vi "decodeStream.vi"(8 "error in (no error)":errorcluster, 9 "beginIndex":i32, 10 "binary stream":u8[](array[numeric]), 11 "tBSONDocumentElement in":refnum<class "tBSONDocumentElement.lvclass">) -> (0 "error out":errorcluster, 1 "endIndex":i32, 2 "binary stream out":u8[](array[numeric]), 3 "tBSONDocumentElement out":refnum<class "tBSONDocumentElement.lvclass">)   [LabVIEW 2013, in "BSON.lvlib" / "tBSONDocumentElement.lvclass"]
uses:
  tBSONDocumentElement.lvclass
  tBSONElement/tBSONElement.lvclass
  setValue.vi
  tBSONDocument/tBSONDocument.lvclass
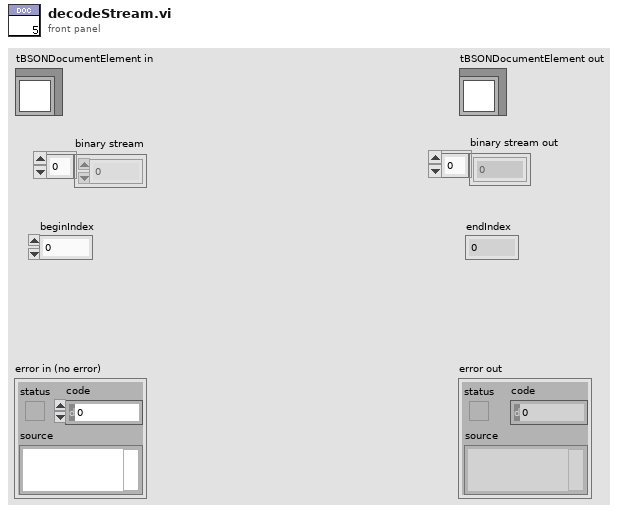
[diagram p1: front panel]
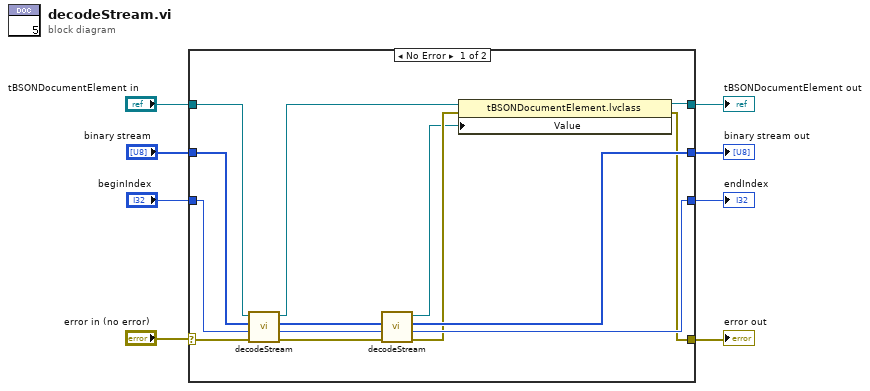
[diagram p0: block diagram]
diagram:
  n1 = case shown="No Error" "error in (no error)" {
    selector: "error in (no error)" -> [w22 w23]
    tunnel: "beginIndex" -> [w19 w24]
    tunnel: "binary stream" -> [w20 w25]
    tunnel: "tBSONDocumentElement in" -> [w21 w26]
    tunnel: [w12 w26] -> w4
    tunnel: [w15 w25] -> w3
    tunnel: [w14 w24] -> w2
    tunnel: [w10 w23] -> w1
    frame No Error {
      n2 = call-parent "decodeStream.vi"("error in (no error)"=w22, "beginIndex"=w19, "binary stream"=w20, "tBSONElement in"=w21) -> ("error out"=w16:errorcluster, "endIndex"=w17:i32, "binary stream out"=w18:u8[], "tBSONElement out"=w13:refnum<class "tBSONDocumentElement.lvclass">)  [unwired: 4 in]
      n3 = call "decodeStream.vi"("error in (no error)"=w16, "Begin Index"=w17, "Byte Data In"=w18) -> ("error out"=w11:errorcluster, "End Index"=w14:i32, "Byte Data Out"=w15:u8[], "tBSONDocument out"=w9:refnum<class "tBSONDocument.lvclass">)  [unwired: 5 in]
      n4 = property class="tBSONDocumentElement.lvclass"(reference=w13, error in=w11, "Value"=w9) -> (reference out=w12:refnum<class "tBSONDocumentElement.lvclass">, error out=w10:errorcluster)
    }
    frame Error {
    }
  }
  "error out" <- w1
  "tBSONDocumentElement out" <- w4
  "binary stream out" <- w3
  "endIndex" <- w2
